vi "Default Data.vi"(2 "Num Rows":i32, 3 "TestMenu in":refnum<class "TestMenu.lvclass">) -> (0 "Default Data":string[][](table), 1 "TestMenu out":refnum<class "TestMenu.lvclass">)   [LabVIEW 2013, in "TestMenu.lvclass"]
doc: "Fill existing rows with 0's, unless specifically overridden."
uses:
  TestMenu.lvclass
  ColumnVIs/MenuCol/MenuCol.lvclass
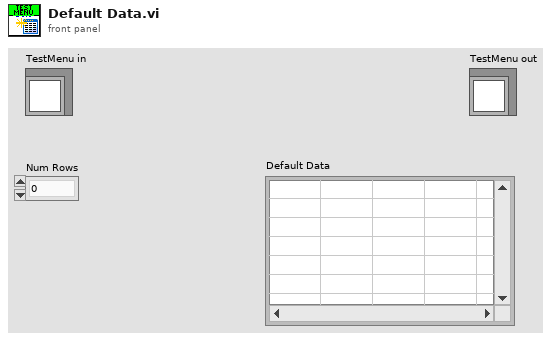
[diagram p1: front panel]
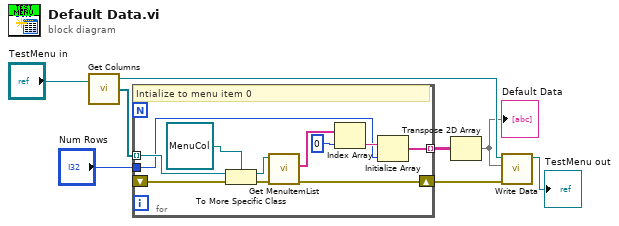
[diagram p0: block diagram]
diagram:
  n1 = call-dynamic "Get Columns.vi"("Device in"="TestMenu in") -> ("Device out"=w6:refnum<class "TestMenu.lvclass">, "Columns"=w5:refnum<class "Column.lvclass">[])  [unwired: 1 in, 1 out]
  n2 = for {
    tunnel: w5 -> [w18] mode=indexing
    shift-right: [w14] -> w4
    shift-left: _ -> [w15]
    tunnel: "Num Rows" -> [w10]
    tunnel: [w9] -> w2 mode=indexing
    # "Intialize to menu item 0"
    n3 = To More Specific Class(target class=refnum<class "MenuCol.lvclass"> refnum ("MenuCol.lvclass"), reference=w18, error in=w15) -> (specific class reference=w17:refnum<class "MenuCol.lvclass">, error out=w19:errorcluster)
    n4 = call-dynamic "Get MenuItemList.vi"("error in (no error)"=w19, "MenuCol in"=w17) -> ("error out"=w14:errorcluster, "MenuItemList"=w13:string[])  [unwired: 7 in, 1 out]
    n5 = Index Array(array=w13, index=0) -> (element=w11:string)
    n6 = Initialize Array(w11, w10) -> (w9:string[])
  }
  n7 = Transpose 2D Array(2D array=w2) -> (transposed array=w1:string[][])
  "Default Data" <- w1
  n8 = call-dynamic "Write Data.vi"("error in (no error)"=w4, "Data"=w1, "Device in"=w6) -> ("Device Out"=→"TestMenu out":refnum<class "TestMenu.lvclass">)  [unwired: 7 in, 1 out]
